vi "Convert Column to Field.vi"(8 "error in (no error)":errorcluster, 10 "Field Configuration":refnum<class "Field Configuration.lvclass">, 11 "Basic Form in":refnum<class "Basic Form.lvclass">) -> (0 "error out":errorcluster, 3 "Basic Form out":refnum<class "Basic Form.lvclass">)   [LabVIEW 2020, in "Form.lvlib" / "Basic Form.lvclass"]
uses:
  Basic Form.lvclass
  C:/Users/User/Desktop/Raman Program/Database OOP/source/Database OOP/Table Libraries/Basic Table/Basic Table Class/Basic Table.lvclass
  Column Libraries/Basic Fields/Field Configurations/Field Configuration Class/Field Configuration.lvclass
  C:/Users/User/Desktop/Raman Program/Database OOP/source/Database OOP/Column Libraries/Basic Columns/Column Configuration/Basic Column Configuration Class/Column Configuration.lvclass
  Column Libraries/Composed Field/Composed Field.lvclass
  C:/Users/User/Desktop/Raman Program/Database OOP/source/Database OOP/Column Libraries/Column Interface/Column Interface Class/Column Interface.lvclass
  Column Libraries/Column/Composed Column.lvclass
  Basic Table/Basic Table Class/Basic Table.lvclass/Basic Table.ctl
  Basic Form.lvclass/Basic Form.ctl
  Table Configuration Interface/Table Configuration Interface.lvclass
  Column Libraries/Basic Columns/Column Configuration/Column Factory Parent Class/Column Factory.lvclass
  Basic Table/Basic Table Class/Basic Table.lvclass
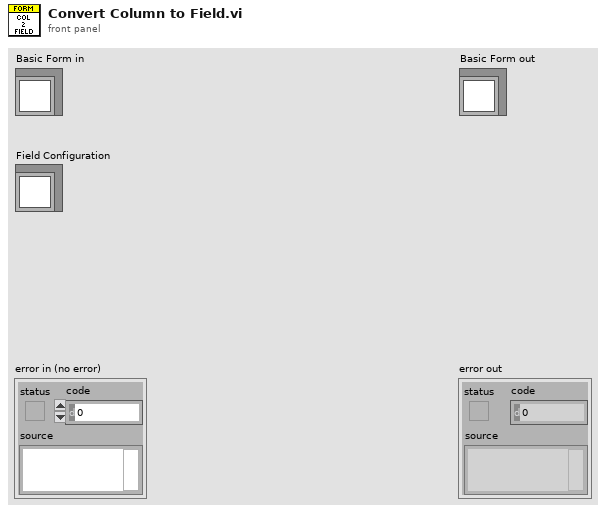
[diagram p1: front panel]
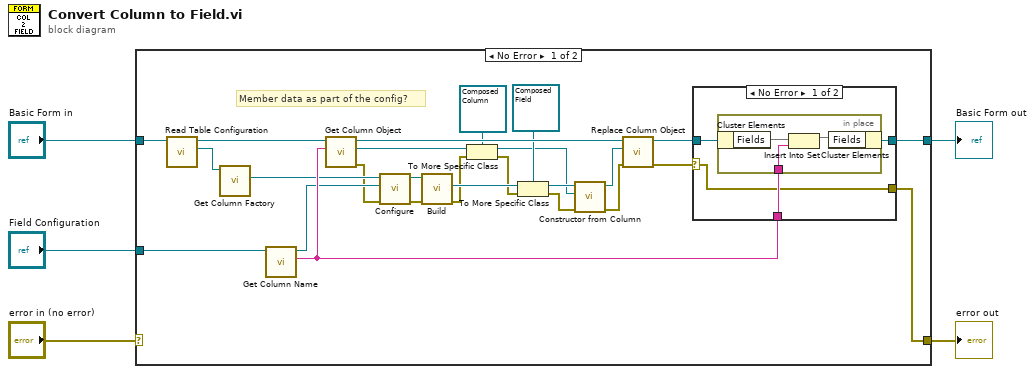
[diagram p0: block diagram]
diagram:
  n1 = case shown="No Error" "error in (no error)" {
    selector: "error in (no error)" -> [_ w42]
    tunnel: [w27 w42] -> w4
    tunnel: [w28 w41] -> w2
    tunnel: "Basic Form in" -> [w24 w41]
    tunnel: "Field Configuration" -> [w26 _]
    frame No Error {
      # "Member data as part of the config?"
      n2 = call "Read Table Configuration.vi"("Basic Table in"=w24) -> ("Table Configuration"=w22:refnum<class "Table Configuration Interface.lvclass">, "Basic Table out"=w23:refnum<class "Basic Form.lvclass">)  [unwired: 8 in, 1 out]
      n3 = call-dynamic "Get Column Factory.vi"("Table Configuration Interface in"=w22) -> ("Column Factory"=w21:refnum<class "Column Factory.lvclass">)  [unwired: 8 in, 2 out]
      n4 = call-dynamic "Get Column Name.vi"("Basic Column Configuration in"=w26) -> ("Column Name"=w25:string, "Basic Column Configuration out"=w20:refnum<class "Field Configuration.lvclass">)  [unwired: 8 in, 1 out]
      n5 = call "Get Column Object.vi"("Column Name"=w25, "Table in"=w23) -> ("error out"=w18:errorcluster, "Column Object"=w12:refnum<class "Column Interface.lvclass">, "Table out"=w31:refnum<class "Basic Form.lvclass">)  [unwired: 7 in]
      n6 = call-dynamic "Configure.vi"("error in (no error)"=w18, "Configuration"=w20, "Column Factory in"=w21) -> ("error out"=w17:errorcluster, "Column Factory out"=w19:refnum<class "Column Factory.lvclass">)  [unwired: 7 in]
      n7 = call-dynamic "Build.vi"("error in (no error)"=w17, "Column Factory in"=w19) -> ("error out"=w8:errorcluster, "Column"=w14:refnum<class "Column Interface.lvclass">)  [unwired: 7 in, 1 out]
      n8 = To More Specific Class(target class=refnum<class "Composed Column.lvclass"> refnum ("Composed Columns.lvlib:Composed Column.lvclass"), reference=w12, error in=w8) -> (specific class reference=w10:refnum<class "Composed Column.lvclass">, error out=w7:errorcluster)
      n9 = To More Specific Class(target class=refnum<class "Composed Field.lvclass"> refnum ("Composed Fields.lvlib:Composed Field.lvclass"), reference=w14, error in=w7) -> (specific class reference=w13:refnum<class "Composed Field.lvclass">, error out=w16:errorcluster)
      n10 = call "Constructor from Column.vi"("error in (no error)"=w16, "Column"=w10, "Composed Field in"=w13) -> ("error out"=w6:errorcluster, "Composed Field out"=w9:refnum<class "Composed Field.lvclass">)  [unwired: 7 in]
      n11 = call "Replace Column Object.vi"("error in (no error)"=w6, "Column Object"=w9, "Table in"=w31) -> ("error out"=w30:errorcluster, "Table out"=w29:refnum<class "Basic Form.lvclass">)  [unwired: 7 in]
      n12 = case shown="No Error" w30 {
        selector: w30 -> [w32 w39]
        tunnel: w29 -> [w35 w40]
        tunnel: w25 -> [w34 _]
        tunnel: [w33 w40] -> w28
        tunnel: [w32 w39] -> w27
        frame No Error {
          n13 = in-place {
            in-place-border: w34 -> [w36]
            n14 = in-place-cluster #1(w35) -> ("Fields"=w38:set{string})
            n15 = Insert Into Set(10:w36, 11:w38) -> (3:w37:set{string})  [unwired: 1 out]
            n16 = in-place-cluster #1("Fields"=w37) -> (w33:refnum<class "Basic Form.lvclass">)
          }
        }
        frame Error {
        }
      }
    }
    frame Error {
    }
  }
  "error out" <- w4
  "Basic Form out" <- w2
